vi "Git-Enterprise-Register Git Client with Authentication.vi"(8 "error in (no error)":errorcluster, 11 "Postman Hash":string) -> (0 "error out":errorcluster, 3 "Refnum out":T1)   [LabVIEW 2020]
uses:
  <vilib>/httpClient/ClientHandle.ctl
  <vilib>/httpClient/LabVIEWHTTPClient.lvlib
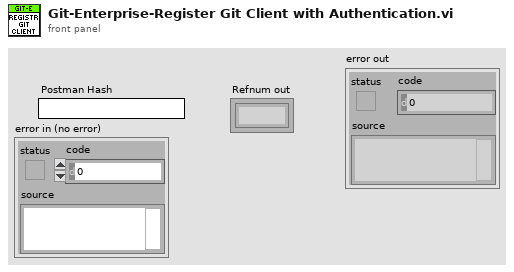
[diagram p1: front panel]
types:
  T1 = typedef "LabVIEWHTTPClient.lvlib/ClientHandle.ctl" = refnum<k1>
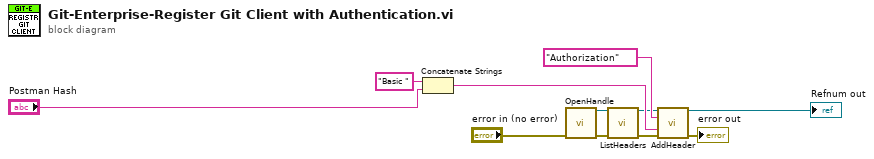
[diagram p0: block diagram]
diagram:
  n1 = Concatenate Strings("Basic " ("string"), "Postman Hash") -> (w11:string)
  n2 = call <vilib>:"OpenHandle.vi"("error in (no error)"="error in (no error)") -> ("client handle out"=w3:T1, "error out"=w4:errorcluster)  [unwired: 13 in]
  n3 = call <vilib>:"ListHeaders.vi"("client handle"=w3, "error in (no error)"=w4) -> ("client handle out"=w5:T1, "error out"=w6:errorcluster)  [unwired: 11 in, 1 out]
  n4 = call <vilib>:"AddHeader.vi"("client handle"=w5, "header"="Authorization", "value"=w11, "error in (no error)"=w6) -> ("client handle out"=→"Refnum out":T1, "error out"=→"error out":errorcluster)  [unwired: 10 in]
